vi "Menu Selection (User).vi"(8 "error in (no error)":errorcluster, 9 "ItemPath":string, 10 "ItemTag":string, 11 "Shortcut Menu in":refnum<class "Shortcut Menu.lvclass">) -> (0 "error out":errorcluster, 3 "Shortcut Menu out":refnum<class "Shortcut Menu.lvclass">)   [LabVIEW 2021, in "Shortcut Menu.lvlib" / "Shortcut Menu.lvclass"]
doc: "Menu Selection (User).vi"
uses:
  <userlib>/John_Lib/Interfaces/Shortcut Menu/Shortcut Menu.lvclass
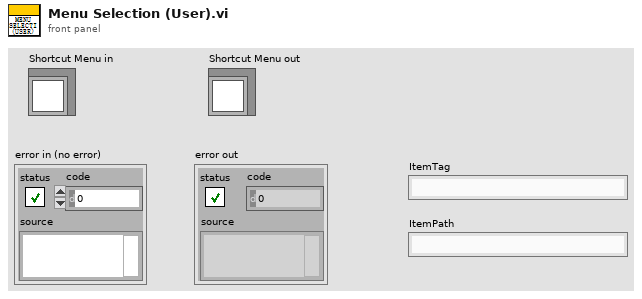
[diagram p1: front panel]
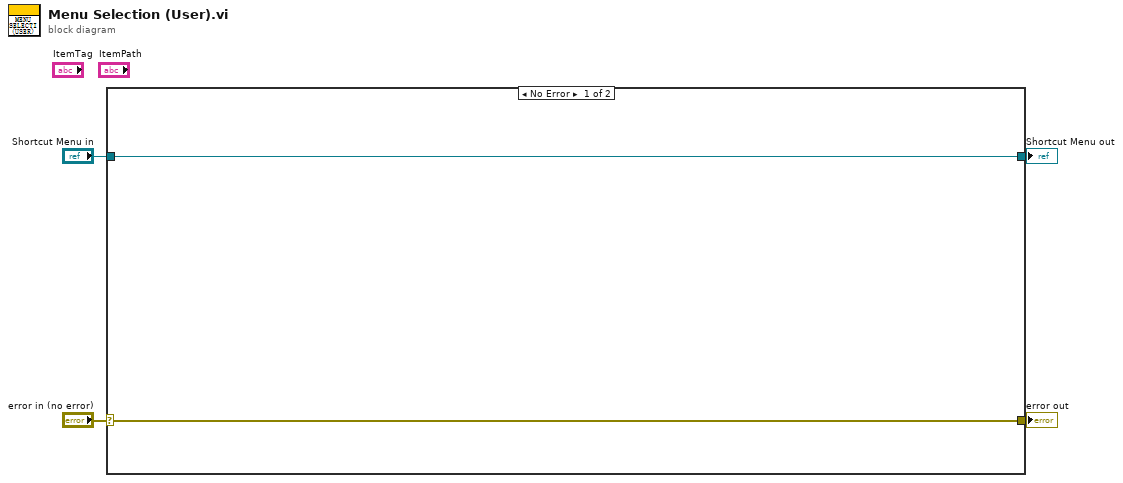
[diagram p0: block diagram]
diagram:
  n1 = case shown="No Error" "error in (no error)" {
    selector: "error in (no error)" -> [w5 w8]
    tunnel: [w5 w8] -> w3
    tunnel: [w6 w7] -> w1
    tunnel: "Shortcut Menu in" -> [w6 w7]
    frame No Error {
    }
    frame Error {
    }
  }
  "error out" <- w3
  "Shortcut Menu out" <- w1
